vi "Interface.vi"() -> ()   [LabVIEW 2020]
panel:
  in  "Test Information":T1 {"Time Stamp" format="%<%H:%M\n%d/%m/%Y>T"; "Operator" items=["Dan McClurg", "Jason Rall", "Laura Vickers", "Daniel Henscheid", "Dwayne Pierce", "Hannah Morrison", "Charles Reyes", "GUEST"]}
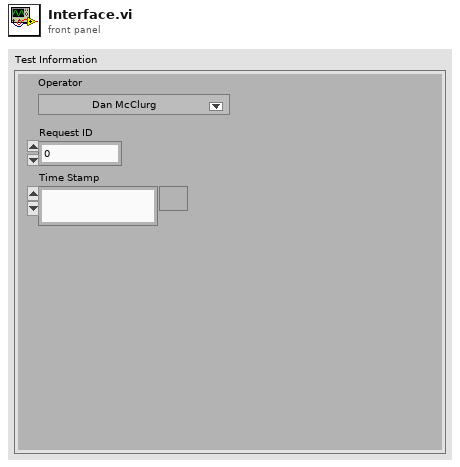
[diagram p1: front panel]
types:
  T1 = cluster{"Operator":u16, "Request ID":i32, "Time Stamp":timestamp}
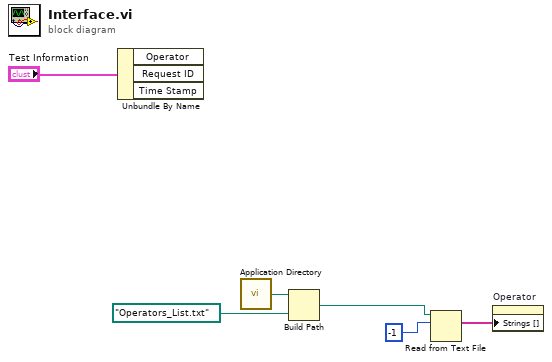
[diagram p0: block diagram]
diagram:
  n1 = Unbundle By Name("Test Information") -> ()  [unwired: 3 out]
  n2 = call <vilib>:"Application Directory.vi"() -> ("Application Directory"=w5:path)
  n3 = Build Path(base path=w5, name or relative path=path "Operators_List.txt" ("file (use dialog)")) -> (appended path=w3:path)
  n4 = Read from Text File(file (use dialog)=w3, count=-1) -> (text=w1:string[])  [unwired: 2 in, 3 out]
  n5 = property on="Operator" class="Ring (strict)"("Strings []"=w1) -> ()  [unwired: 2 in, 2 out]
